vi "poly_dialog_interrupt_1btn.vi"(8 "error in":errorcluster caption="Error in (no error)", 9 "button name (\"OK\")":string="OK", 10 "message":string) -> (0 "error out":errorcluster)   [LabVIEW 2015]
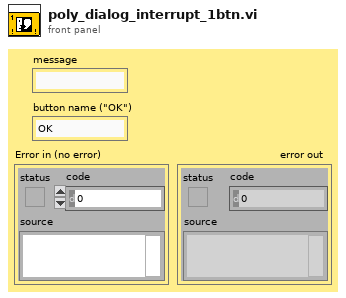
[diagram p1: front panel]
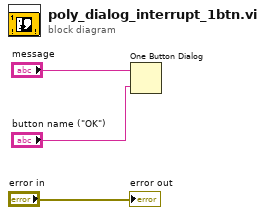
[diagram p0: block diagram]
diagram:
  n1 = One Button Dialog(message="message", button name ("OK")="button name (\"OK\")") -> ()  [unwired: 1 out]
  "error out" <- "error in"
